vi "Cleanup.vi"(8 "error in (no error)":errorcluster, 11 "App in":refnum<class "App.lvclass">) -> (0 "error out":errorcluster)   [LabVIEW 2020, in "PicoG-App.lvlib" / "App.lvclass"]
uses:
  App.lvclass
  App.lvclass/App.ctl
  <vilib>/IlluminatedG/IG OOPanel/OOPanel/Manager/Manager.lvclass
  App Watcher/App Watcher.lvclass
  Builds/picoG/ppl/PicoG-Core.lvlibp/PicoG-Processor/PicoG-Core/PlatformPluginManager/PlatformPluginManager.lvclass
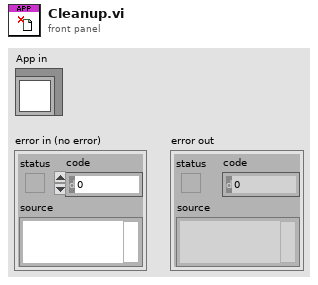
[diagram p1: front panel]
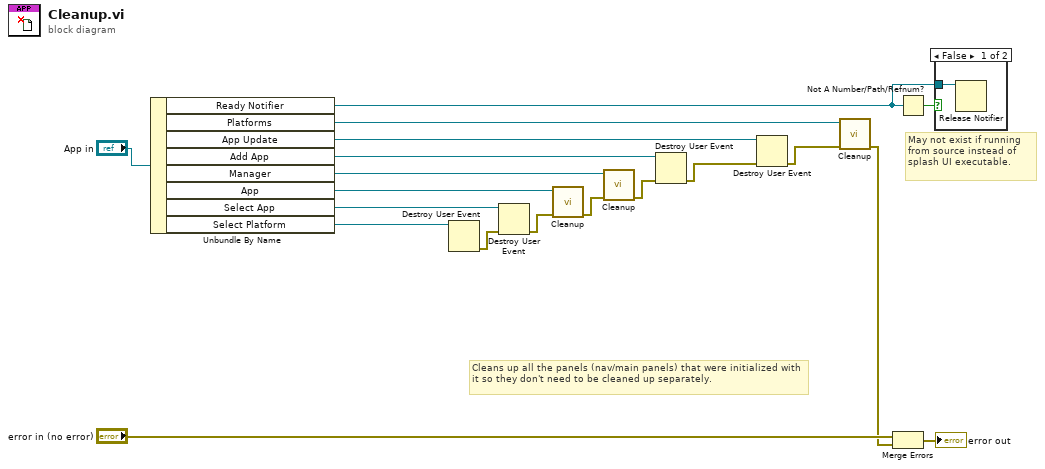
[diagram p0: block diagram]
diagram:
  # "May not exist if running from source instead of splash UI executable."
  # "Cleans up all the panels (nav/main panels) that were initialized with it so they don't need to be cleaned up separately."
  n1 = Unbundle By Name("App in") -> ("Ready Notifier"=w9:refnum<notifier>, "Platforms"=w12:refnum<class "PlatformPluginManager.lvclass">, "App Update"=w7:refnum<user-event>, "Add App"=w16:refnum<user-event>, "Manager"=w17:refnum<class "Manager.lvclass">, "App"=w14:refnum<class "App Watcher.lvclass">, "Select App"=w4:refnum<user-event>, "Select Platform"=w5:refnum<user-event>)
  n2 = Destroy User Event(user event=w5) -> (error out=w3:errorcluster)  [unwired: 1 in]
  n3 = Destroy User Event(user event=w4, error in=w3) -> (error out=w2:errorcluster)
  n4 = call <vilib>:"Cleanup.vi"("error in (no error)"=w2, "App Watcher in"=w14) -> ("error out"=w13:errorcluster)  [unwired: 9 in]
  n5 = call <vilib>:"Cleanup.vi"("error in (no error)"=w13, "Manager in"=w17) -> ("error out"=w15:errorcluster)  [unwired: 7 in, 2 out]
  n6 = Destroy User Event(user event=w16, error in=w15) -> (error out=w1:errorcluster)
  n7 = Destroy User Event(user event=w7, error in=w1) -> (error out=w6:errorcluster)
  n8 = call <vilib>:"Cleanup.vi"("error in (no error)"=w6, "TargetPluginManager in"=w12) -> ("error out"=w10:errorcluster)  [unwired: 9 in]
  n9 = Merge Errors("error in (no error)", w10) -> (→"error out":errorcluster)
  n10 = Not A Number/Path/Refnum?(number/path/refnum=w9) -> (NaN/Path/Refnum?=w8:bool)
  n11 = case shown="False" w8 {
    tunnel: w9 -> [w20 _]
    frame False {
      n12 = Release Notifier(notifier=w20) -> ()  [unwired: 2 in, 3 out]
    }
    frame True {
    }
  }
